vi "Uart Get Channels.vi"(8 "error in (no error)":errorcluster, 11 "LINX Client in":refnum<class "LINX Client.lvclass">) -> (0 "error out":errorcluster, 1 "Names":string[](array[string]), 2 "Channels":u8[](array[numeric]), 3 "LINX Client out":refnum<class "LINX Client.lvclass">)   [LabVIEW 2020, in "LINX Client.lvclass"]
uses:
  LINX Client.lvclass
  LINX Base.lvclass
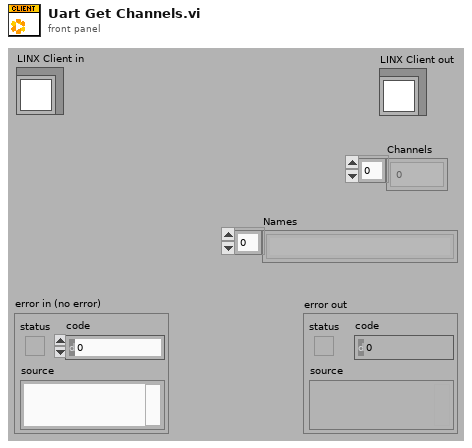
[diagram p1: front panel]
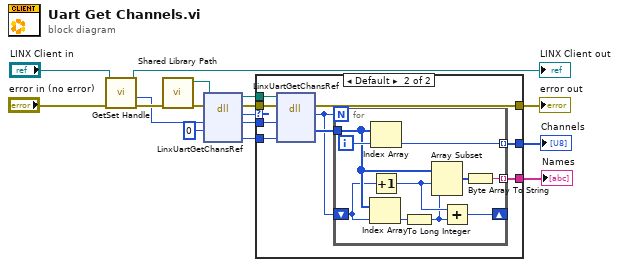
[diagram p0: block diagram]
diagram:
  n1 = call-dynamic "GetSet Handle.vi"("error in"="error in (no error)", "LINX Base in"="LINX Client in") -> ("error out"=w4:errorcluster, "handle out"=w1:u64, "LINX Base out"=→"LINX Client out":refnum<class "LINX Client.lvclass">)  [unwired: 3 in, 4 out]
  n2 = call "Shared Library Path.vi"("error in (no error)"=w4) -> ("error out"=w15:errorcluster, "Path"=w16:path)  [unwired: 9 out]
  n3 = dll-call lib="Z:/Development/LabVIEW Hobbyist Toolkit/LabVIEW/vi.lib/MakerHub/LINX/Resources/libLinxDevice.dll" fn="LinxUartGetChansRef"(path in=w16, error in=w15, "device"=w1, "buffer"=u64 0) -> (path out=w9:path, error out=w10:errorcluster, "numDevs"=w11:i32, "device"=w12:u64, "bytes"=w13:u32)  [unwired: 1 in, 2 out]
  n4 = case shown="Default" w11 {
    tunnel: w13 -> [_ w26]
    tunnel: w12 -> [_ w25]
    tunnel: w10 -> [w17 w24]
    tunnel: w9 -> [_ w23]
    tunnel: [w17 w22] -> w8
    tunnel: [_ w19] -> w7
    tunnel: [_ w18] -> w6
    frame 0 {
    }
    frame Default {
      n5 = dll-call lib="Z:/Development/LabVIEW Hobbyist Toolkit/LabVIEW/vi.lib/MakerHub/LINX/Resources/libLinxDevice.dll" fn="LinxUartGetChansRef"(path in=w23, error in=w24, "device"=w25, "bytes"=w26) -> (error out=w22:errorcluster, "numDevs"=w20:i32, "buffer"=w21:u8[])  [unwired: 3 in, 2 out]
      n6 = for {
        N: w20 -> [_]
        tunnel: w21 -> [w35]
        shift-right: [w31] -> _
        shift-left: w20 -> [w34]
        tunnel: [w29] -> w18 mode=indexing
        tunnel: [w27] -> w19 mode=indexing
        i -> [w36]
        n7 = Index Array(array=w35, index=w34) -> (element=w32:u8)
        n8 = Index Array(array=w35, index=w36) -> (element=w29:u8)
        n9 = Increment(x=w34) -> (x+1=w33:i32)
        n10 = To Long Integer(number=w32) -> (32bit integer=w30:i32)
        n11 = Array Subset(array=w35, index=w33, length=w30) -> (w28:u8[])
        n12 = Add(x=w33, y=w30) -> (x+y=w31:i32)
        n13 = Byte Array To String(unsigned byte array=w28) -> (string=w27:string)
      }
    }
  }
  "error out" <- w8
  "Names" <- w7
  "Channels" <- w6
